vi "Get Static I64.vi"(6 "Write?":bool, 8 "error in (no error)":errorcluster, 9 "Tag":string, 10 "Value Type":refnum<class "Abs_I64 Integer.lvclass">, 11 "Var Bus in":refnum<class "Omni_Bus.lvclass">) -> (0 "error out":errorcluster, 2 "Value Out":refnum<class "Abs_I64 Integer.lvclass">, 3 "Var Bus out":refnum<class "Omni_Bus.lvclass">)   [LabVIEW 2021, in "Omni_Bus.lvclass"]
uses:
  Omni_Bus.lvclass
  Omni_Bus.lvclass/Omni_Bus.ctl
  <vilib>/TSA/Abstract Data Classes/Abs_Types/I64 Integer/Abs_I64 Integer.lvclass
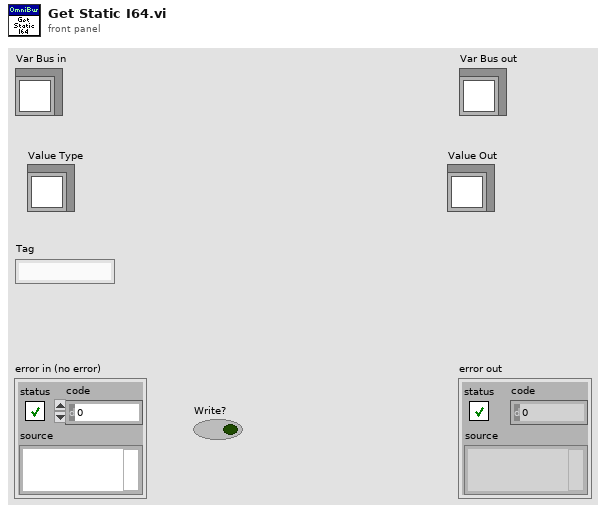
[diagram p1: front panel]
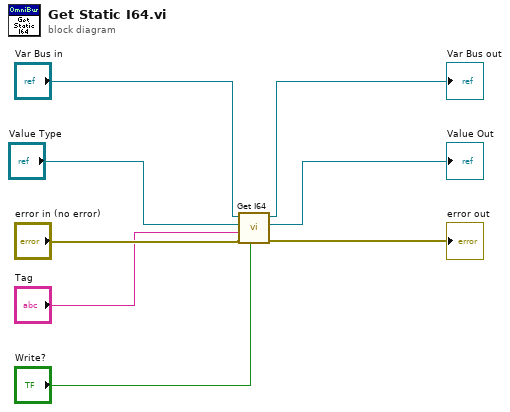
[diagram p0: block diagram]
diagram:
  n1 = call-dynamic "Get I64.vi"("Write?"="Write?", "error in (no error)"="error in (no error)", "Tag"="Tag", "Value Type"="Value Type", "Var Bus in"="Var Bus in") -> ("error out"=→"error out":errorcluster, "Value Out"=→"Value Out":refnum<class "Abs_I64 Integer.lvclass">, "Var Bus out"=→"Var Bus out":refnum<class "Omni_Bus.lvclass">)  [unwired: 4 in]
